vi "VFD_Pump_Run.vi"(7 "PWM Frequency [Hz]":dbl=10000.0, 9 "Pump speed (%)":dbl=1.0 min=1.0 max=99.0) -> (3 "task out":refnum<k21>)   [LabVIEW 2021]
uses:
  Human_Labview/global_variables.vi
  <vilib>/DAQmx/create/channels.llb/DAQmx Create Channel (CO-Pulse Generation-Frequency).vi
  <vilib>/DAQmx/configure/timing.llb/DAQmx Timing (Implicit).vi
  <resource>/objmgr/daqmx.rc
panel:
  out "Actual Duty Cycle 2":dbl=0.99
  out "Actual Freq 2":dbl=200.0
  out "[PWM Duty Cycle %]\nPUMP Speed Analog \nVoltage Control":dbl(slide)=99.0 scale=0.0..100.0
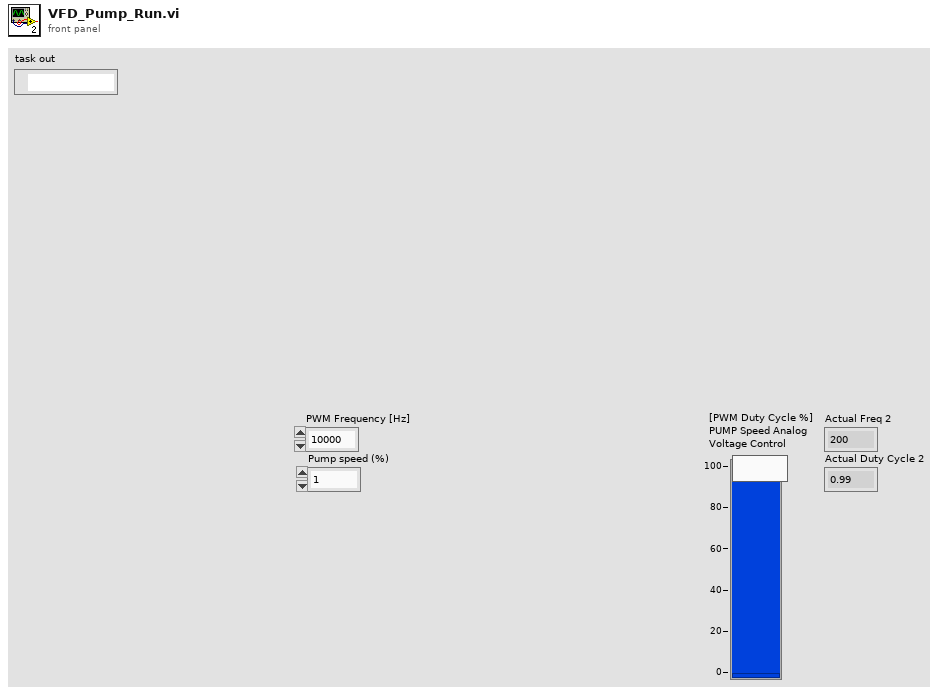
[diagram p1: front panel]
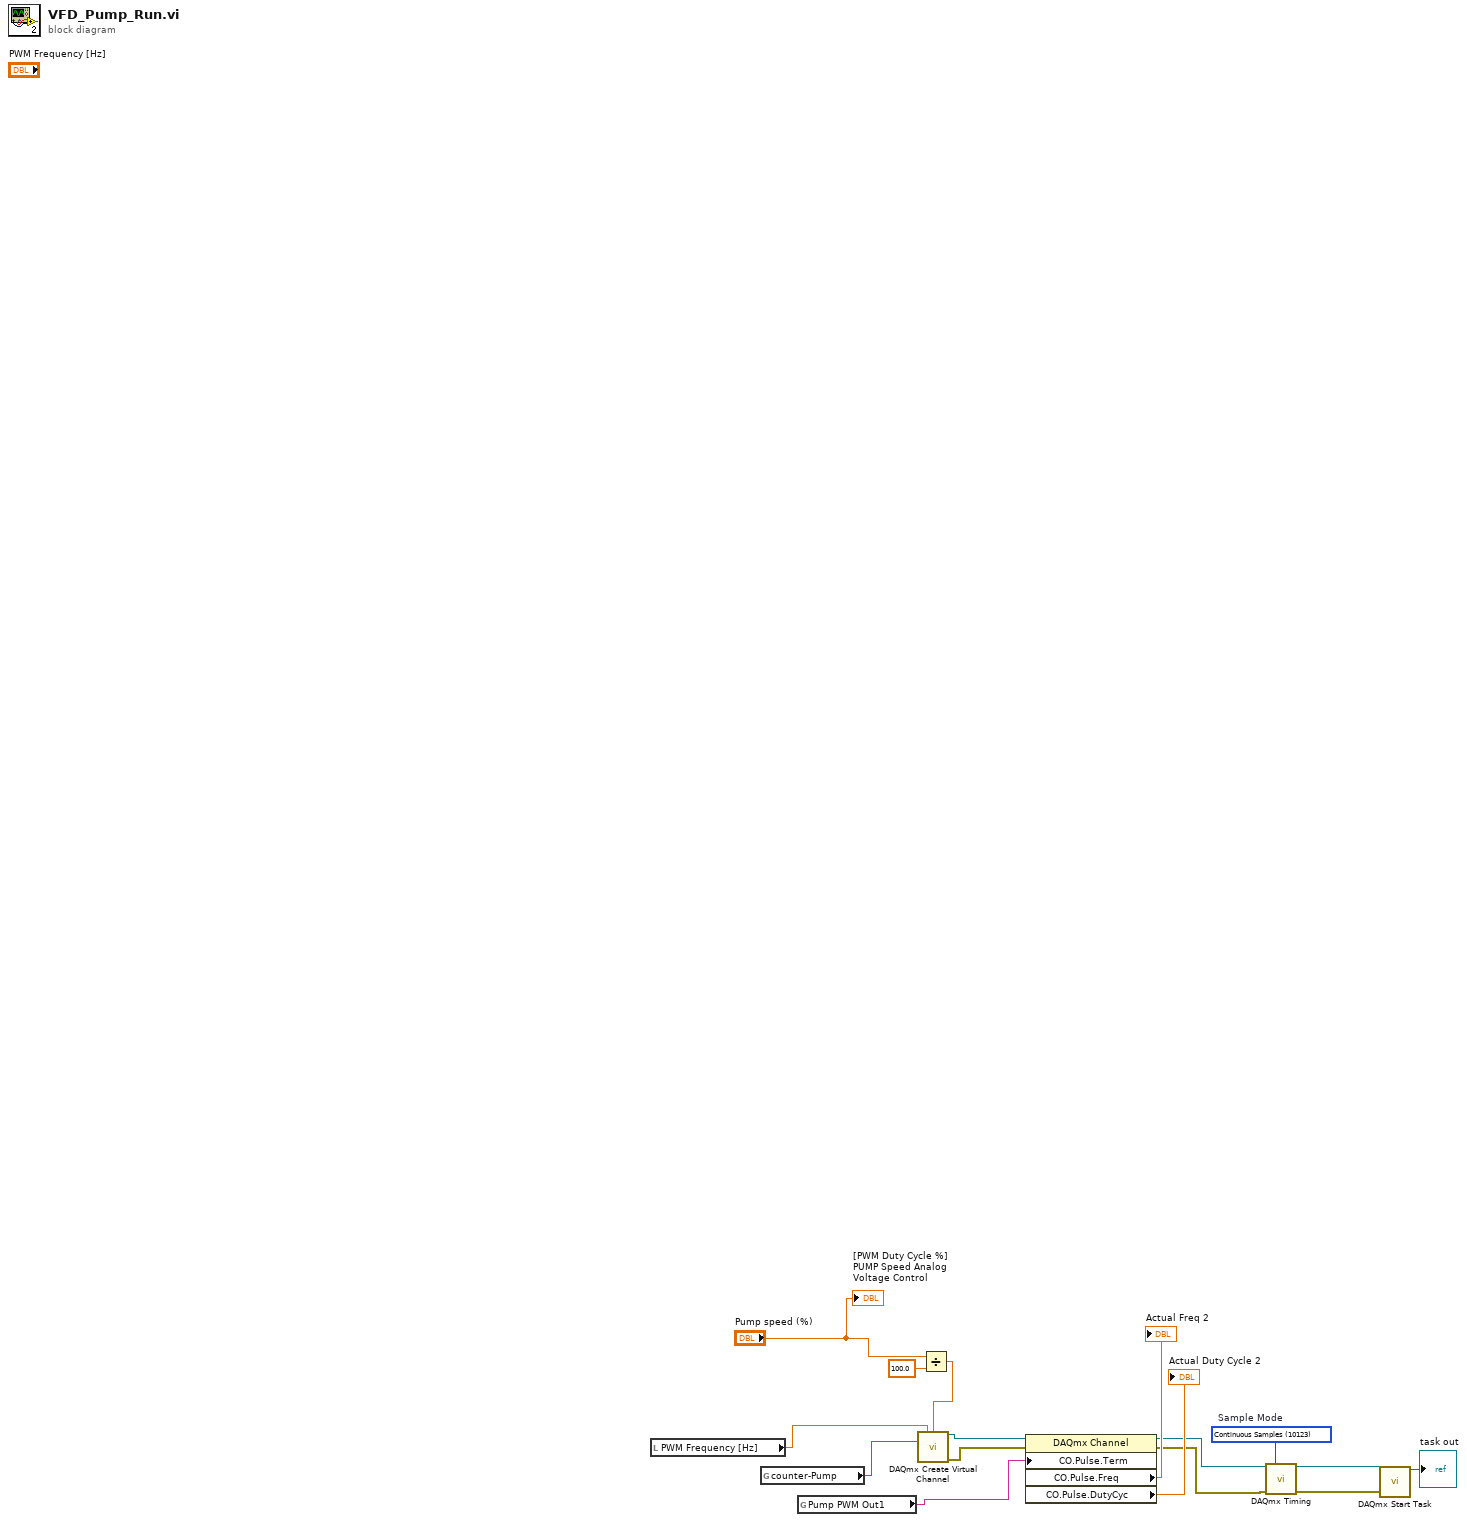
[diagram p0: block diagram]
diagram:
  w4 = 10123 items=["Finite Samples"=10178, "Continuous Samples"=10123, "Hardware Timed Single Point"=12522]  # Sample Mode
  n1 = local read "PWM Frequency [Hz]"() -> (w2:dbl)
  n2 = global read "global_variables.vi" "counter-Pump"() -> (w15:tag)
  n3 = global read "global_variables.vi" "Pump PWM Out1"() -> (w16:tag)
  n4 = Divide(x="Pump speed (%)", y=100.0) -> (x/y=w13:dbl)
  n5 = call-poly <vilib>:"DAQmx Create Virtual Channel.vi"("frequency"=w2, "duty cycle"=w13, "counter"=w15) -> ("task out"=w10:refnum<k21>, "error out"=w9:errorcluster)  [unwired: 11 in]
  n6 = property class="DAQmx Channel"(reference=w10, error in=w9, "CO.Pulse.Term"=w16) -> (reference out=w8:refnum<k21>, error out=w7:errorcluster, "CO.Pulse.Freq"=→"Actual Freq 2":dbl, "CO.Pulse.DutyCyc"=→"Actual Duty Cycle 2":dbl)
  n7 = call-poly <vilib>:"DAQmx Timing.vi"("task/channels in"=w8, "sample mode"=w4, "error in"=w7) -> ("task out"=w5:refnum<k21>, "error out"=w6:errorcluster)  [unwired: 11 in]
  n8 = call <vilib>:"DAQmx Start Task.vi"("task/channels in"=w5, "error in"=w6) -> ("task out"=→"task out":refnum<k21>)  [unwired: 12 in, 1 out]
  "[PWM Duty Cycle %]\nPUMP Speed Analog \nVoltage Control" <- "Pump speed (%)"
